vi "Create Utility.vi"(8 "error in (no error)":errorcluster, 11 "Device Item Ref in":T1 format="%.0x") -> (0 "error out":errorcluster)   [LabVIEW 2020, in "G5 Regatron Custom Device System Explorer.lvlib"]
uses:
  G5 Regatron Custom Device System Explorer.lvlib
  <vilib>/NI VeriStand/Custom Device API/Custom Device Item Ref.ctl
  <vilib>/NI VeriStand/Custom Device API/Custom Device Channel.ctl
  <vilib>/NI VeriStand/Custom Device API/Custom Device Channel Type.ctl
  <vilib>/NI VeriStand/Custom Device API/Custom Device API.lvlib
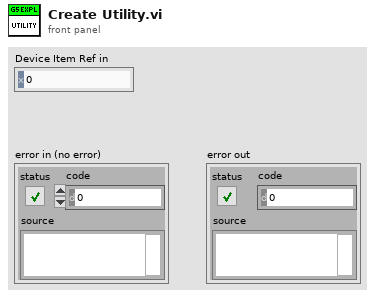
[diagram p1: front panel]
types:
  T1 = typedef "Custom Device API.lvlib/Custom Device Item Ref.ctl" = u64
  T2 = typedef "Custom Device API.lvlib/Custom Device Channel.ctl" = cluster{"Type":T3, "Units":string, "Default Value":dbl, "Faultable":bool, "Scalable":bool}
  T3 = typedef "Custom Device API.lvlib/Custom Device Channel Type.ctl" = enum16{"Input", "Output"}
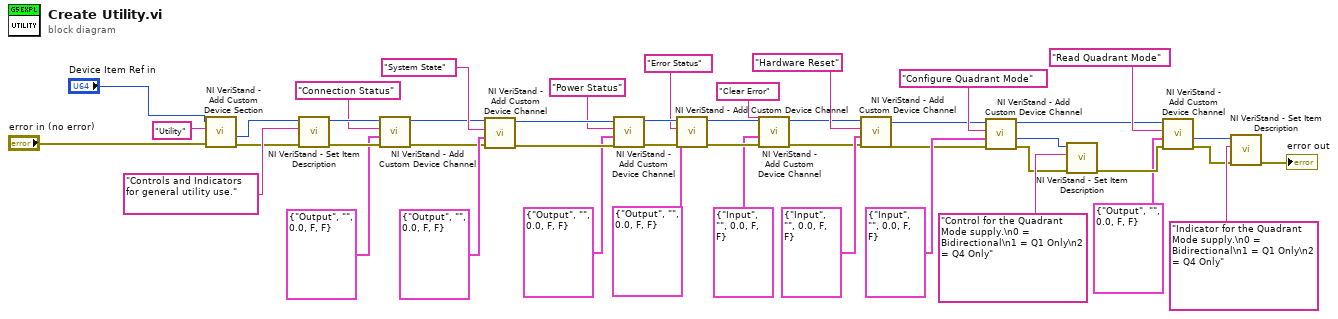
[diagram p0: block diagram]
diagram:
  n1 = call <vilib>:"NI VeriStand - Add Custom Device Section.vi"("error in (no error)"="error in (no error)", "Section Name"="Utility", "Parent Ref in"="Device Item Ref in") -> ("error out"=w34:errorcluster, "Section Ptr"=w33:T1)  [unwired: 5 in, 2 out]
  n2 = call <vilib>:"NI VeriStand - Set Item Description.vi"("error in (no error)"=w34, "Description"="Controls and Indicators for general utility use.", "Item Ref in"=w33) -> ("error out"=w36:errorcluster, "Item Ref out"=w35:T1)  [unwired: 6 in, 1 out]
  n3 = call <vilib>:"NI VeriStand - Add Custom Device Channel.vi"("error in (no error)"=w36, "Channel"=T2 {"Type"=enum."Output", "Units"="", "Default Value"=0.0, "Faultable"=FALSE, "Scalable"=FALSE}, "Channel Name"="Connection Status", "Parent Ref in"=w35) -> ("error out"=w17:errorcluster, "Parent Ref out"=w15:T1)  [unwired: 4 in, 2 out]
  n4 = call <vilib>:"NI VeriStand - Add Custom Device Channel.vi"("error in (no error)"=w17, "Channel"=T2 {"Type"=enum."Output", "Units"="", "Default Value"=0.0, "Faultable"=FALSE, "Scalable"=FALSE}, "Channel Name"="System State", "Parent Ref in"=w15) -> ("error out"=w18:errorcluster, "Parent Ref out"=w16:T1)  [unwired: 4 in, 2 out]
  n5 = call <vilib>:"NI VeriStand - Add Custom Device Channel.vi"("error in (no error)"=w18, "Channel"=T2 {"Type"=enum."Output", "Units"="", "Default Value"=0.0, "Faultable"=FALSE, "Scalable"=FALSE}, "Channel Name"="Power Status", "Parent Ref in"=w16) -> ("error out"=w9:errorcluster, "Parent Ref out"=w7:T1)  [unwired: 4 in, 2 out]
  n6 = call <vilib>:"NI VeriStand - Add Custom Device Channel.vi"("error in (no error)"=w9, "Channel"=T2 {"Type"=enum."Output", "Units"="", "Default Value"=0.0, "Faultable"=FALSE, "Scalable"=FALSE}, "Channel Name"="Error Status", "Parent Ref in"=w7) -> ("error out"=w10:errorcluster, "Parent Ref out"=w8:T1)  [unwired: 4 in, 2 out]
  n7 = call <vilib>:"NI VeriStand - Add Custom Device Channel.vi"("error in (no error)"=w10, "Channel"=T2 {"Type"=enum."Input", "Units"="", "Default Value"=0.0, "Faultable"=FALSE, "Scalable"=FALSE}, "Channel Name"="Clear Error", "Parent Ref in"=w8) -> ("error out"=w21:errorcluster, "Parent Ref out"=w22:T1)  [unwired: 4 in, 2 out]
  n8 = call <vilib>:"NI VeriStand - Add Custom Device Channel.vi"("error in (no error)"=w21, "Channel"=T2 {"Type"=enum."Input", "Units"="", "Default Value"=0.0, "Faultable"=FALSE, "Scalable"=FALSE}, "Channel Name"="Hardware Reset", "Parent Ref in"=w22) -> ("error out"=w26:errorcluster, "Parent Ref out"=w25:T1)  [unwired: 4 in, 2 out]
  n9 = call <vilib>:"NI VeriStand - Add Custom Device Channel.vi"("error in (no error)"=w26, "Channel"=T2 {"Type"=enum."Input", "Units"="", "Default Value"=0.0, "Faultable"=FALSE, "Scalable"=FALSE}, "Channel Name"="Configure Quadrant Mode", "Parent Ref in"=w25) -> ("error out"=w38:errorcluster, "Channel Ref"=w39:T1, "Parent Ref out"=w29:T1)  [unwired: 4 in, 1 out]
  n10 = call <vilib>:"NI VeriStand - Set Item Description.vi"("error in (no error)"=w38, "Description"="Control for the Quadrant Mode supply.\n0 = Bidirectional\n1 = Q1 Only\n2 = Q4 Only", "Item Ref in"=w39) -> ("error out"=w40:errorcluster)  [unwired: 6 in, 2 out]
  n11 = call <vilib>:"NI VeriStand - Add Custom Device Channel.vi"("error in (no error)"=w40, "Channel"=T2 {"Type"=enum."Output", "Units"="", "Default Value"=0.0, "Faultable"=FALSE, "Scalable"=FALSE}, "Channel Name"="Read Quadrant Mode", "Parent Ref in"=w29) -> ("error out"=w42:errorcluster, "Channel Ref"=w44:T1)  [unwired: 4 in, 2 out]
  n12 = call <vilib>:"NI VeriStand - Set Item Description.vi"("error in (no error)"=w42, "Description"="Indicator for the Quadrant Mode supply.\n0 = Bidirectional\n1 = Q1 Only\n2 = Q4 Only", "Item Ref in"=w44) -> ("error out"=→"error out":errorcluster)  [unwired: 6 in, 2 out]
